vi "Initialize.vi"(0 "QCS in":refnum<class "QCS.lvclass">, 5 "HW Address":u32, 11 "error in (no error)":errorcluster) -> (4 "QCS out":refnum<class "QCS.lvclass">, 6 "Instrument ID":string, 15 "error out":errorcluster)   [LabVIEW 2013, in "QCS.lvclass"]
uses:
  Lib.llb/QCS.lvclass
  Lib.llb/CS.lvclass
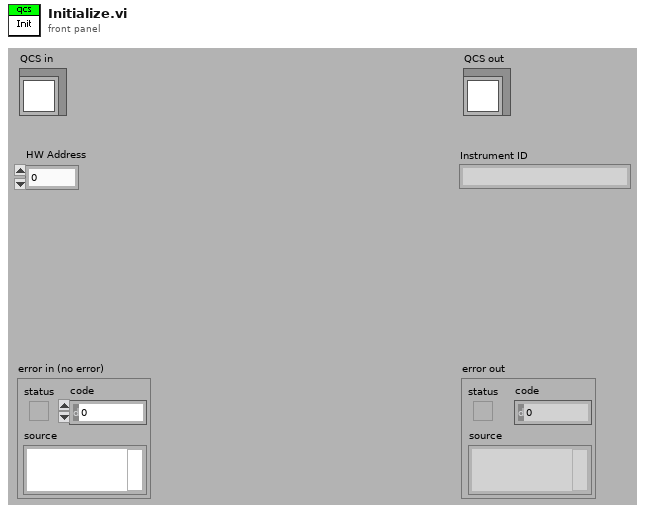
[diagram p1: front panel]
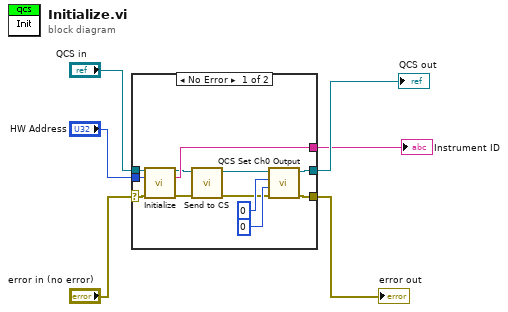
[diagram p0: block diagram]
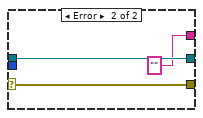
[diagram p2: hidden frame]
diagram:
  n1 = case shown="No Error" "error in (no error)" {
    selector: "error in (no error)" -> [w15 w20]
    tunnel: "QCS in" -> [w18 w21]
    tunnel: [w14 w21] -> w5
    tunnel: "HW Address" -> [w17 _]
    tunnel: [w16 "" ("Instrument ID")] -> w3
    tunnel: [w13 w20] -> w2
    frame No Error {
      n2 = call-parent "Initialize.vi"("CS in"=w18, "HW Address"=w17, "error in (no error)"=w15) -> ("CS out"=w10:refnum<class "QCS.lvclass">, "Instrument ID"=w16:string, "error out"=w8:errorcluster)  [unwired: 10 in]
      n3 = call-dynamic "Send to CS.vi"("error in (no error)"=w8, "QCS in"=w10) -> ("error out"=w7:errorcluster, "QCS out"=w9:refnum<class "QCS.lvclass">)  [unwired: 8 in]
      n4 = call "QCS Set Ch0 Output.vi"("error IO"=w7, "New Channel"=u8 0 ("Old Channel"), "Old Channel"=u8 0, "QCS in"=w9) -> ("error out"=w13:errorcluster, "QCS out"=w14:refnum<class "QCS.lvclass">)  [unwired: 2 out]
    }
    frame Error {
    }
  }
  "error out" <- w2
  "QCS out" <- w5
  "Instrument ID" <- w3
